vi "y_unit_offset.vi"(0 "spectrum y unit (mW pwr absolute)":T1=enum."mW pwr absolute") -> (14 "yUnit val":i32)   [LabVIEW 2010, in "OSA.lvclass"]
doc: "SubVI to a <B>Thorlabs_OSA_64</B> object.\n\n[GOOP 1.0]"
uses:
  OSA.lvclass
  typeDef/spectrum_y_unit.ctl
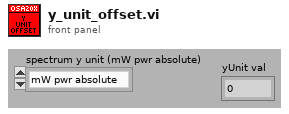
[diagram p1: front panel]
types:
  T1 = typedef "OSA.lvclass/spectrum_y_unit.ctl" = enum16{"dBm pwr absolute", "dBm pwr density", "mW pwr absolute", "mW pwr density"}
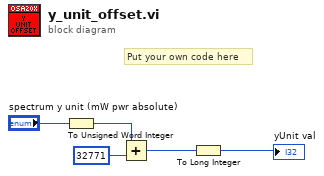
[diagram p0: block diagram]
diagram:
  # "Put your own code here"
  n1 = To Unsigned Word Integer(number="spectrum y unit (mW pwr absolute)") -> (unsigned 16bit integer=w4:u16)
  n2 = Add(x=w4, y=u16 32771) -> (x+y=w2:u16)
  n3 = To Long Integer(number=w2) -> (32bit integer=→"yUnit val":i32)
